vi "Run Script_Meas DC V.vi"(0 "Semiconductor Module Context":T3, 1 "SMU Settings":T2={"Level"=0.0, "Level Range"=0.01, "Limit"=5.0, "Limit Range"=6.0, "Sense"=1009} {"Sense" items=["Local"=1008, "Remote"=1009]}, 2 "script name":string="SoiBG", 5 "Published Data Ids":string[](array[string])=["RF1-DCv"], 7 "Pins":string[](array[string])=["RF1"], 11 "error in (no error)":errorcluster) -> (15 "error Out":errorcluster)   [LabVIEW 2013]
uses:
  <vilib>/NI_TestStand_SemiconductorModule/NI_TestStand_Semiconductor_Module.lvlibp/PinMap/General/SemiconductorModuleContext.ctl
  <instrlib>/niDCPower/nidcpower.llb/niDCPower Sense.ctl
  <instrlib>/niHSDIO/niHSDIO.llb/niHSDIO_ctl Trigger Script - trigID Values (Ring).ctl
  <vilib>/NI_TestStand_SemiconductorModule/NI_TestStand_Semiconductor_Module.lvlibp/PinMap/DC Power/PinsToNIDCPowerSessions.vi
  <vilib>/NI_TestStand_SemiconductorModule/NI_TestStand_Semiconductor_Module.lvlibp/PinMap/General/Publish/PublishDataDouble2D.vi
  <vilib>/NI_TestStand_SemiconductorModule/NI_TestStand_Semiconductor_Module.lvlibp
panel:
  out "Vdc_Array":dbl[][](array[numeric]) format="%#_6p"
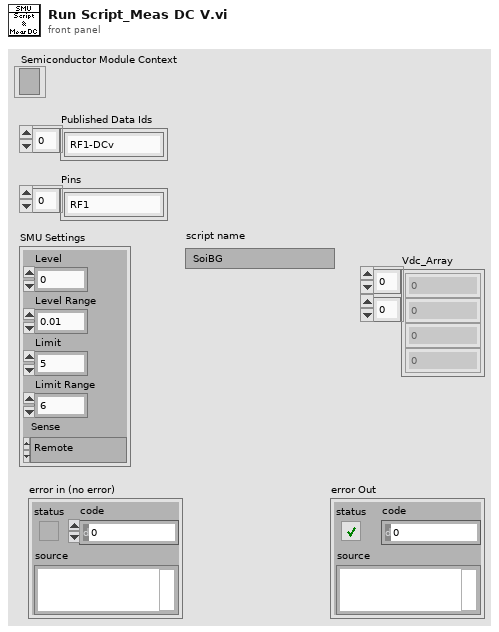
[diagram p1: front panel]
types:
  T1 = typedef "niDCPower Sense.ctl" = i32
  T2 = cluster{"Level":dbl, "Level Range":dbl, "Limit":dbl, "Limit Range":dbl, "Sense":T1}
  T3 = typedef "NI_TestStand_Semiconductor_Module.lvlibp/SemiconductorModuleContext.ctl" = refnum<k7>
  T4 = typedef "niHSDIO_ctl Trigger Script - trigID Values (Ring).ctl" = string
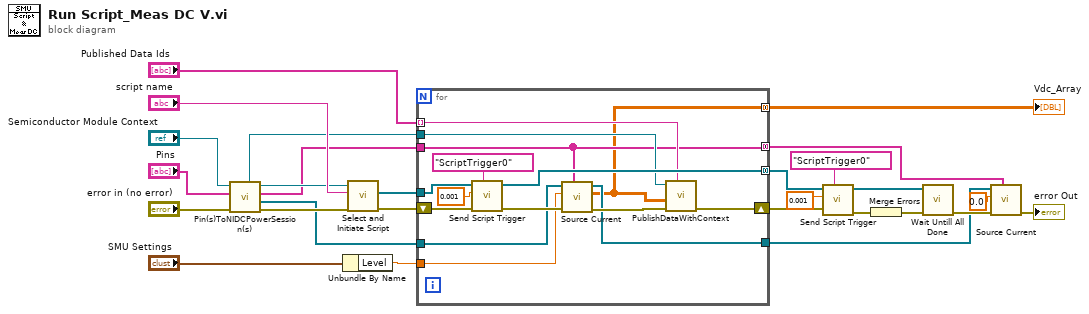
[diagram p0: block diagram]
diagram:
  n1 = call-poly <vilib>:"Pin(s)ToNIDCPowerSession(s).vi"("error in (no error)"="error in (no error)", "Pins"="Pins", "Semiconductor Module Context"="Semiconductor Module Context") -> ("error out"=w15:errorcluster, "Instrument Sessions"=w10:refnum<k15>[], "Channel Lists"=w11:string[], "Semiconductor Module Context Out"=w13:T3, "Pin Query Context"=w7:refnum<class "MultiplePinMultipleSessionQueryContext.lvclass">)  [unwired: 4 in]
  n2 = Unbundle By Name("SMU Settings") -> ("Level"=w8:dbl)
  n3 = call "Select and Initiate Script.vi"("error in (no error)"=w15, "script name"="script name", "Semiconductor Module Context"=w13) -> ("error out"=w27:errorcluster, "HSDIO GEN Sessions Out"=w26:refnum<k15>[])  [unwired: 6 in, 1 out]
  n4 = for {
    tunnel: w26 -> [w41]
    tunnel: "Published Data Ids" -> [w33] mode=indexing
    tunnel: [w39] -> w19 mode=concatenating
    shift-right: [w34] -> w20
    shift-left: w27 -> [w42]
    tunnel: w11 -> [w29]
    tunnel: w10 -> [w36]
    tunnel: w8 -> [w32]
    tunnel: w7 -> [w31]
    tunnel: [w30] -> w4
    tunnel: [w29] -> w2 mode=concatenating
    tunnel: [w28] -> w1 mode=concatenating
    n5 = call "Send Script Trigger.vi"("trigger id (script trigger 0)"=T4 "ScriptTrigger0", "error in (no error)"=w42, "Delay Time (s)"=0.001, "HSDIO Sessions In"=w41) -> ("error out"=w37:errorcluster, "HSDIO Sessions Out"=w39:refnum<k15>[])  [unwired: 6 in]
    n6 = call "Source Current.vi"("Channel Lists"=w29, "error in (no error)"=w37, "current level"=w32, "Instrument Sessions In"=w36) -> ("error out"=w35:errorcluster, "voltage measurements"=w28:dbl[][], "Instrument Sessions Out"=w30:refnum<k15>[])  [unwired: 4 in, 1 out]
    n7 = call-poly <vilib>:"PublishDataWithContext.vi"("Published Data Id"=w33, "error in (no error)"=w35, "Data In"=w28, "Pin Query Context"=w31) -> ("error out"=w34:errorcluster)  [unwired: 6 in, 1 out]
  }
  "Vdc_Array" <- w1
  n8 = call "Send Script Trigger.vi"("trigger id (script trigger 0)"=T4 "ScriptTrigger0", "error in (no error)"=w20, "Delay Time (s)"=0.001, "HSDIO Sessions In"=w19) -> ("error out"=w21:errorcluster, "HSDIO Sessions Out"=w18:refnum<k15>[])  [unwired: 6 in]
  n9 = Merge Errors(w21) -> (w23:errorcluster)
  n10 = call "Wait Untill All Done.vi"("error in (no error)"=w23, "HSDIO Sessions In"=w18) -> ("error out"=w6:errorcluster)  [unwired: 8 in, 1 out]
  n11 = call "Source Current.vi"("Channel Lists"=w2, "error in (no error)"=w6, "current level"=0.0, "Instrument Sessions In"=w4) -> ("error out"=→"error Out":errorcluster)  [unwired: 4 in, 3 out]
